vi "Write DIO.vi"(8 "error in (no error)":errorcluster, 10 "FIU Engine Refs in":T1 {"RT IDs"."Slot #" max=15; "RT IDs"."Chip Address (A2 A1 A0)" max=7; "RT Block Data Refs"."Data Reference" format="%.0x"}, 11 "DMA FIFO Ref in":refnum<k20>) -> (0 "error out":errorcluster, 2 "FIU Engine Refs out":T1 {"RT IDs"."Slot #" max=15; "RT IDs"."Chip Address (A2 A1 A0)" max=7; "RT Block Data Refs"."Data Reference" format="%.0x"})   [LabVIEW 2014, in "SLSC configuration Engine.lvlib"]
uses:
  SLSC configuration Engine.lvlib
  Type Defs/RT Engine Refs.ctl
  Shared/Type Defs/RT IDs.ctl
  Shared/SPI Utility/Slot #.ctl
  Shared/MCP23S17/Chip Address.ctl
  <vilib>/NI Veristand/Custom Device API/Block Data Reference.ctl
  <vilib>/NI Veristand/Custom Device API/Data Reference.ctl
  <vilib>/NI Veristand/Custom Device API/Global Data Refs.vi
  <vilib>/NI Veristand/Custom Device API/Custom Device API.lvlib
  Shared/SLSC configuration Shared.lvlib
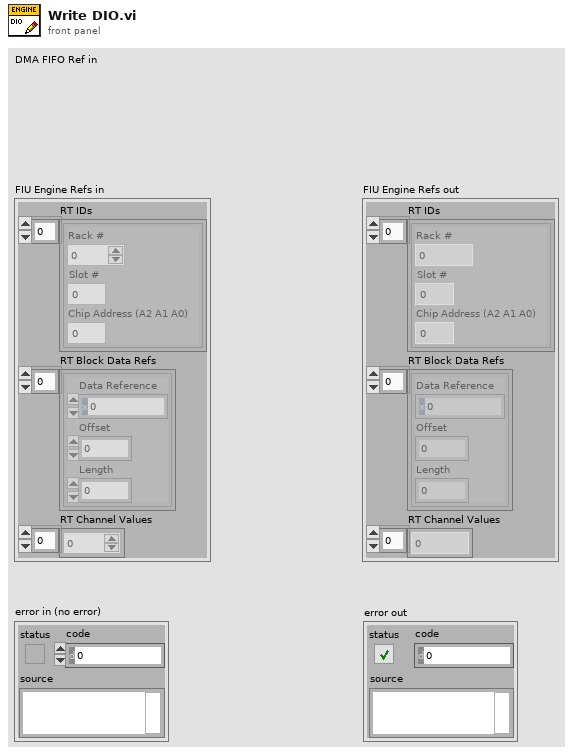
[diagram p1: front panel]
types:
  T1 = typedef "SLSC configuration Engine.lvlib/RT Engine Refs.ctl" = cluster{"RT IDs":T2[], "RT Block Data Refs":T5[], "RT Channel Values":dbl[]}
  T2 = typedef "SLSC configuration Shared.lvlib/RT IDs.ctl" = cluster{"Rack #":u8, "Slot #":T3, "Chip Address (A2 A1 A0)":T4}
  T3 = typedef "SLSC configuration Shared.lvlib/Slot #.ctl" = u8
  T4 = typedef "SLSC configuration Shared.lvlib/Chip Address.ctl" = u8
  T5 = typedef "Custom Device API.lvlib/Block Data Reference.ctl" = cluster{"Data Reference":T6, "Offset":i32, "Length":i32}
  T6 = typedef "Custom Device API.lvlib/Data Reference.ctl" = i32
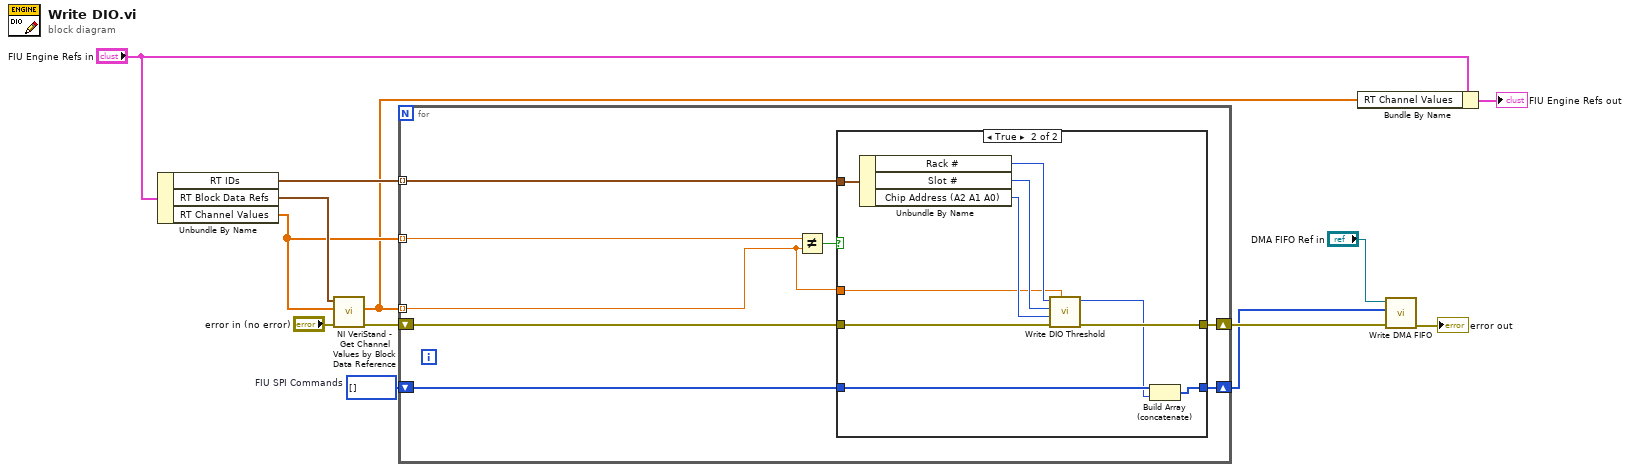
[diagram p0: block diagram]
diagram:
  w5 = u64[] []  # FIU SPI Commands
  n1 = Unbundle By Name("FIU Engine Refs in") -> ("RT IDs"=w10:T2[], "RT Block Data Refs"=w13:T5[], "RT Channel Values"=w8:dbl[])
  n2 = call <vilib>:"NI VeriStand - Get Channel Values by Block Data Reference.vi"("error in (no error)"="error in (no error)", "Values Array in"=w8, "Block Data Ref"=w13) -> ("error out"=w11:errorcluster, "Values Array out"=w7:dbl[])  [unwired: 6 in, 1 out]
  n3 = for {
    shift-right: [w19] -> w4
    shift-left: w11 -> [w20]
    tunnel: w10 -> [w21] mode=indexing
    tunnel: w7 -> [w15] mode=indexing
    tunnel: w8 -> [w14] mode=indexing
    shift-right: [w16] -> w2
    shift-left: w5 -> [w17]
    n4 = Not Equal?(x=w14, y=w15) -> (x != y?=w18:bool)
    n5 = case shown="True" w18 {
      tunnel: w21 -> [_ w33]
      tunnel: w20 -> [w23 w32]
      tunnel: w15 -> [_ w24]
      tunnel: [w23 w28] -> w19
      tunnel: w17 -> [w22 w27]
      tunnel: [w22 w25] -> w16
      frame False {
      }
      frame True {
        n6 = Unbundle By Name(w33) -> ("Rack #"=w31:u8, "Slot #"=w30:T3, "Chip Address (A2 A1 A0)"=w29:T4)
        n7 = call "Write DIO Threshold.vi"("Logic Threshold (%)"=w24, "error in (no error)"=w32, "Chip Address (A2 A1 A0)"=w29, "Slot #"=w30, "Rack #"=w31) -> ("error out"=w28:errorcluster, "FIFO SPI Message"=w26:u64)  [unwired: 5 in]
        n8 = Build Array (concatenate)(w27, w26) -> (w25:u64[])
      }
    }
  }
  n9 = Bundle By Name(cluster="FIU Engine Refs in", "RT Channel Values"=w7) -> (→"FIU Engine Refs out":T1)
  n10 = call "Write DMA FIFO.vi"("error in (no error)"=w4, "FIU SPI Commands"=w2, "DMA FIFO Ref in"="DMA FIFO Ref in") -> ("error out"=→"error out":errorcluster)  [unwired: 8 in]
